vi "Rename Label.vi"(8 "error in":errorcluster, 9 "number of DO":u8, 10 "number of AI":u8, 11 "number of AO":u8) -> (0 "error out":errorcluster, 3 "label":T1)   [LabVIEW 2022 SP3]
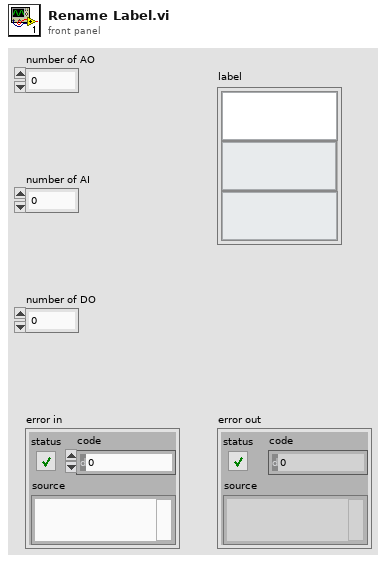
[diagram p1: front panel]
types:
  T1 = cluster{"AO Label":string, "AI Label":string, "DO Label":string}
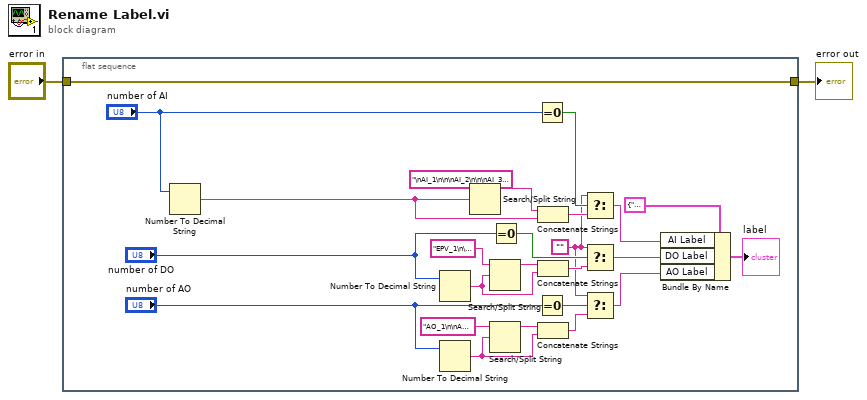
[diagram p0: block diagram]
diagram:
  n1 = flat-sequence {
    tunnel: "error in" -> [w19]
    tunnel: [w19] -> w1
    frame #0 {
      w6 = ""
      n2 = Number To Decimal String(number="number of AI") -> (decimal integer string=w3:string)  [unwired: 1 in]
      n3 = Number To Decimal String(number="number of DO") -> (decimal integer string=w22:string)  [unwired: 1 in]
      n4 = Number To Decimal String(number="number of AO") -> (decimal integer string=w25:string)  [unwired: 1 in]
      n5 = Search/Split String(string="\nAI_1\n\n\nAI_2\n\n\nAI_3\n\n\nAI_4\n\n\nAI_5\n\n\nAI_6\n\n\nAI_7\n\n\nAI_8\n\n\nAI_9\n\n\nAI_10" ("AI Label"), search string/char (-)=w3) -> (substring before match=w24:string)  [unwired: 1 in, 2 out]
      n6 = Search/Split String(string="EPV_1\n\n\nEPV_2\n\n\nEPV_3\n\n\nEPV_4\n\n\nEPV_5\n\n\nEPV_6\n\n\nEPV_7\n\n\nEPV_8\n\n\nEPV_9\n\n\nEPV_10\n\n\n" ("Label"), search string/char (-)=w22) -> (substring before match=w23:string)  [unwired: 1 in, 2 out]
      n7 = Search/Split String(string="AO_1\n\nAO_2\n\nAO_3\n\nAO_4" ("AO Label"), search string/char (-)=w25) -> (substring before match=w27:string)  [unwired: 1 in, 2 out]
      n8 = Equal To 0?(x="number of DO") -> (x = 0?=w12:bool)
      n9 = Equal To 0?(x="number of AI") -> (x = 0?=w15:bool)
      n10 = Equal To 0?(x="number of AO") -> (x = 0?=w8:bool)
      n11 = Concatenate Strings(w24, w3) -> (w14:string)
      n12 = Concatenate Strings(w23, w22) -> (w9:string)
      n13 = Concatenate Strings(w27, w25) -> (w5:string)
      n14 = Select(t=w6, s=w15, f=w14) -> (s? t:f=w13:string)
      n15 = Select(t=w6, s=w12, f=w9) -> (s? t:f=w11:string)
      n16 = Select(t=w6, s=w8, f=w5) -> (s? t:f=w4:string)
      n17 = Bundle By Name(cluster=T1 {"AO Label"="AO_1\n\nAO_2\n\nAO_3", "AI Label"="\nAI_1\n\n\nAI_2\n\n\nAI_3", "DO Label"="EPV_1\n\n\nEPV_2\n\n\nEPV_3"} ("label"), "AI Label"=w13, "DO Label"=w11, "AO Label"=w4) -> (→"label":T1)
    }
  }
  "error out" <- w1
